vi "CRYCurveLib Info Interface.vi"(7 "sAction":string, 10 "sData":string, 11 "sOption":string) -> ()   [LabVIEW 2013]
uses:
  Control/CRYCurveLib Info Cluster.ctl
  Global/CRYCurve Library Global.vi
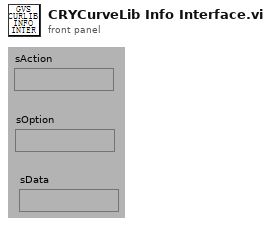
[diagram p1: front panel]
types:
  T1 = cluster{"Section":string, "Item":cluster{"Key":string, "Value":string}[]}
  T2 = typedef "CRYCurveLib Info Cluster.ctl" = cluster{"GroupingState":string}
  T3 = cluster{"Section":string, "Items":cluster{"Key":string, "Value":string}[]}[]
  T4 = cluster{"Section":string, "Items":cluster{"Key":string, "Value":string}[]}
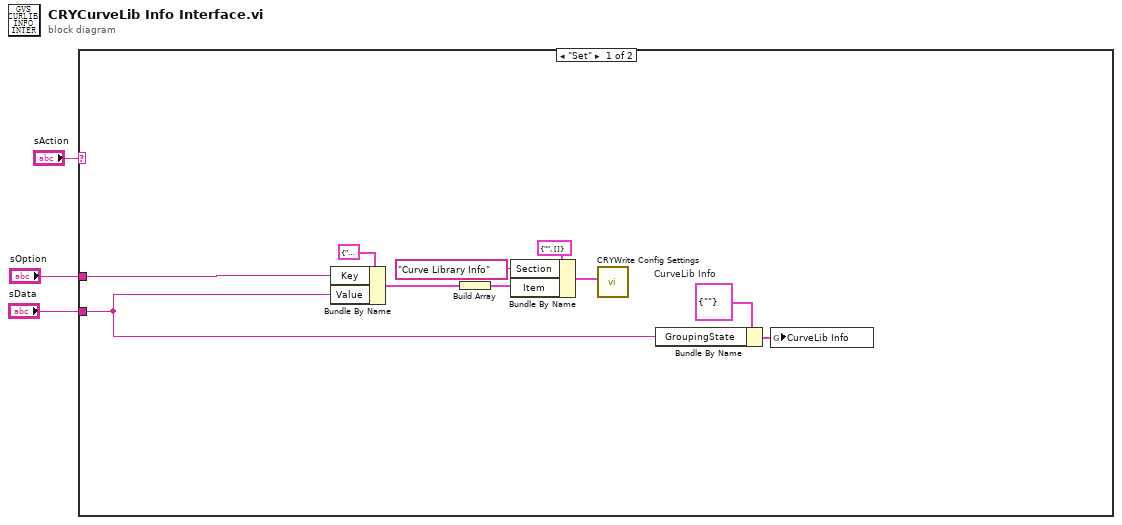
[diagram p0: block diagram]
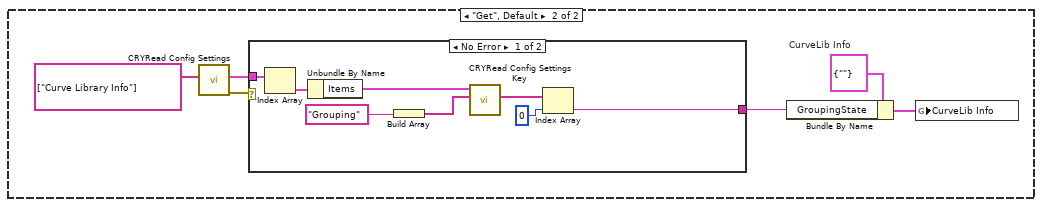
[diagram p2: hidden frame]
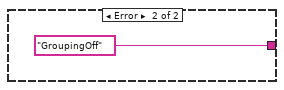
[diagram p3: hidden frame]
diagram:
  n1 = case shown="\"Set\"" "sAction" {
    tunnel: "sOption" -> [w7 _]
    tunnel: "sData" -> [w4 _]
    frame "Set" {
      w6 = T2 {"GroupingState"=""}  # CurveLib Info
      n2 = Bundle By Name(cluster=cluster{"Key":string, "Value":string} {"Key"="", "Value"=""} ("Cluster"), "Key"=w7, "Value"=w4) -> (w12:cluster{"Key":string, "Value":string})
      n3 = Build Array(w12) -> (w11:cluster{"Key":string, "Value":string}[])
      n4 = Bundle By Name(cluster=T1 {"Section"="", "Item"=[]}, "Section"="Curve Library Info", "Item"=w11) -> (w8:T1)
      n5 = call "CRYWrite Config Settings.vi"("Config Data"=w8) -> ()  [unwired: 8 in, 1 out]
      n6 = Bundle By Name(cluster=w6, "GroupingState"=w4) -> (w5:T2)
      n7 = global write "CRYCurve Library Global.vi" "CurveLib Info"(w5) -> ()
    }
    frame "Get", Default {
      w16 = T2 {"GroupingState"=""}  # CurveLib Info
      n8 = call "CRYRead Config Settings.vi"("Section"=string[] ["Curve Library Info"]) -> ("error out"=w19:errorcluster, "Configuration Data"=w18:T3)  [unwired: 9 in]
      n9 = case shown="No Error" w19 {
        tunnel: w18 -> [w27 _]
        tunnel: [w20 "GroupingOff" ("Section")] -> w14
        frame No Error {
          n10 = Index Array(array=w27) -> (element=w26:T4)  [unwired: 1 in]
          n11 = Unbundle By Name(w26) -> ("Items"=w22:cluster{"Key":string, "Value":string}[])
          n12 = Build Array("Grouping" ("Section")) -> (w23:string[])
          n13 = call "CRYRead Config Settings Key.vi"("Key Names"=w23, "Items"=w22) -> ("Values"=w21:string[])  [unwired: 9 in]
          n14 = Index Array(array=w21, index=0) -> (element=w20:string)
        }
        frame Error {
        }
      }
      n15 = Bundle By Name(cluster=w16, "GroupingState"=w14) -> (w15:T2)
      n16 = global write "CRYCurve Library Global.vi" "CurveLib Info"(w15) -> ()
    }
  }
